vi "asset.create.vi"(8 "error in":errorcluster, 9 "Description":string, 10 "Title":string, 11 "Nominal Client in":refnum<class "Nominal Client.lvclass">) -> (0 "error out":errorcluster, 2 "asset":refnum<class "asset.lvclass">, 3 "Nominal Client out":refnum<class "Nominal Client.lvclass">)   [LabVIEW 2020, in "Nominal Client.lvclass"]
doc: "Triggers an ingest job, allowing either creating a new dataset or uploading to an existing one. This endpoint is meant to supersede all other ingestion endpoints as their functionality gets migrated to this one."
uses:
  Nominal Client.lvclass
  asset/asset.lvclass
  Nominal Client.lvclass/Nominal Client.ctl
  nominal types/workspace/workspace.lvclass/workspace.ctl
  workspace.get.vi
  <vilib>/JDP Science/JSONtext/Merge into Object.vi
  workspace.add_to_payload.vi/88650e10-de3e-481c-85db-71cb0fdf4485.vi
  nominal types/workspace/rid.get.vi
  <vilib>/JDP Science/JSONtext/Variant to JSON Text.vi
  <vilib>/JDP Science/JSONtext/Get all Object Items.vi
  <vilib>/JDP Science/JSONtext/Set Multiple Object Items.vi
  <vilib>/JDP Science/JSONtext/LVClass Serializer/JSONtext LVClass Serializer.lvclass
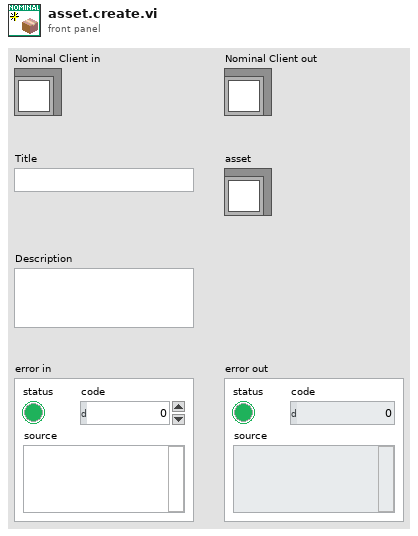
[diagram p1: front panel]
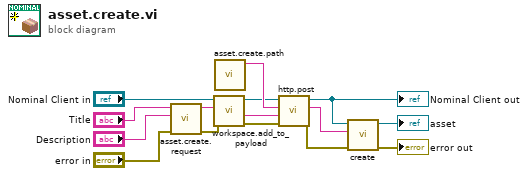
[diagram p0: block diagram]
diagram:
  n1 = call "asset.create.request.vi"("error in"="error in", "Description"="Description", "Title"="Title") -> ("error out"=w2:errorcluster, "request"=w1:string)  [unwired: 7 in]
  n2 = call "workspace.add_to_payload.vi"("error in"=w2, "JSON payload in"=w1, "Nominal Client in"="Nominal Client in") -> ("error out"=w8:errorcluster, "JSON payload out"=w9:string, "Nominal Client out"=w7:refnum<class "Nominal Client.lvclass">)  [unwired: 6 in]
  n3 = call "asset.create.path.vi"() -> ("path"=w10:string)  [unwired: 10 in, 1 out]
  n4 = call "http.post.vi"("error in"=w8, "Request body"=w9, "Path"=w10, "Nominal Client in"=w7) -> ("error out"=w14:errorcluster, "Response"=w15:string, "Nominal Client out"=w11:refnum<class "Nominal Client.lvclass">)  [unwired: 4 in, 1 out]
  "Nominal Client out" <- w11
  n5 = call "create.vi"("error in"=w14, "asset"=w15, "Nominal Client"=w11) -> ("error out"=→"error out":errorcluster, "asset"=→"asset":refnum<class "asset.lvclass">)  [unwired: 7 in]
